vi "Get_Instrument.vi"(8 "error in (no error)":errorcluster caption="entrée d'erreur (pas d'erreur)", 11 "Test (Default) en entrée":refnum<class "Test (Default).lvclass">) -> (0 "error out":errorcluster caption="sortie d'erreur", 2 "Library Instruments.lvlib:Class Instrument (Default).lvclass":refnum<class "Class Instrument (Default).lvclass">, 3 "Test (Default) en sortie":refnum<class "Test (Default).lvclass">)   [LabVIEW 2020, in "Library Test.lvlib" / "Test (Default).lvclass"]
uses:
  Test (Default).lvclass
  Instrument/Instrument (Default)/Class Instrument (Default).lvclass
  Test (Default).lvclass/Test (Default).ctl
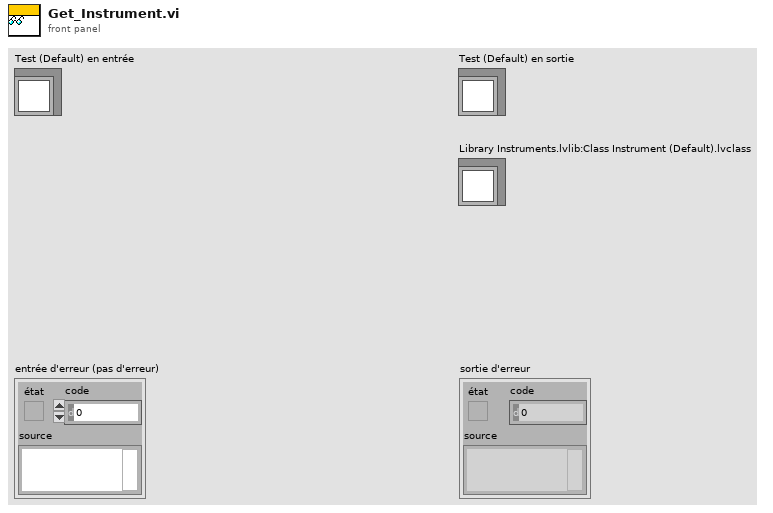
[diagram p1: front panel]
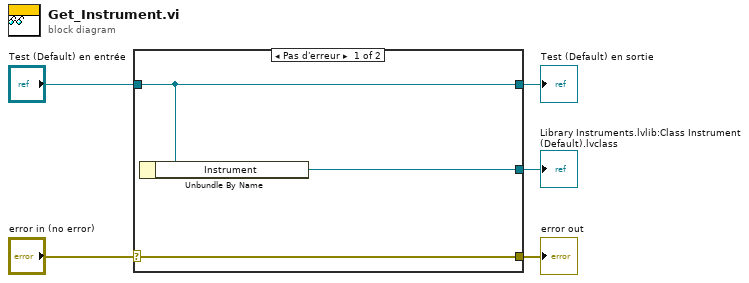
[diagram p0: block diagram]
diagram:
  n1 = case shown="Pas d'erreur" "error in (no error)" {
    selector: "error in (no error)" -> [w8 w9]
    tunnel: [w8 w9] -> w4
    tunnel: [w7 w10] -> w2
    tunnel: "Test (Default) en entrée" -> [w7 w10]
    tunnel: [w6 _] -> w1
    frame No Error {
      n2 = Unbundle By Name(w7) -> ("Instrument"=w6:refnum<class "Class Instrument (Default).lvclass">)
    }
    frame Error {
    }
  }
  "error out" <- w4
  "Test (Default) en sortie" <- w2
  "Library Instruments.lvlib:Class Instrument (Default).lvclass" <- w1
